vi "L1_AdderTest_File_Appender.vi"(0 "Vin":dbl, 1 "file path (dialog if empty)":path, 5 "CH":dbl, 7 "Active Adder":dbl, 9 "DAC Level":dbl=63.0, 11 "Vmeas":dbl, 12 "IPR":dbl, 13 "Digital Output":dbl) -> (6 "appended array":dbl[](array[numeric]), 14 "file path (dialog if empty) 2":path)   [LabVIEW 2012]
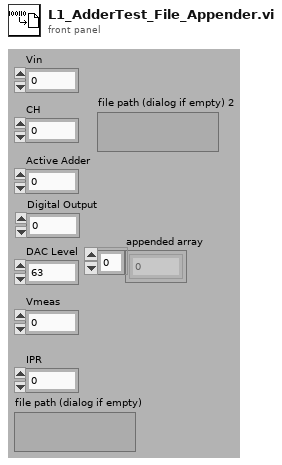
[diagram p1: front panel]
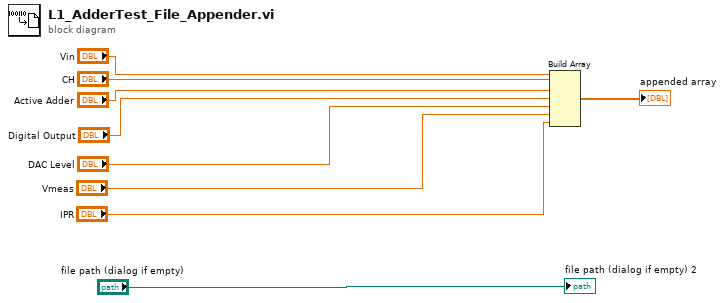
[diagram p0: block diagram]
diagram:
  n1 = Build Array("Vin", "CH", "Active Adder", "Digital Output", "DAC Level", "Vmeas", "IPR") -> (→"appended array":dbl[])
  "file path (dialog if empty) 2" <- "file path (dialog if empty)"
